vi "XML.ListElementTextValuesByCustomQuery.vi"(8 "error in":errorcluster, 10 "XPath expression":string, 11 "XML file path":path=path "C:/Projects/TM-OS/trunk/Design/XML_HW_config2.xml") -> (0 "error out":errorcluster, 2 "values":string[](array[string]))   [LabVIEW 2019, in "Tools.lvlib"]
uses:
  <vilib>/xml/Load XML File.vi
  <vilib>/xml/Close Reference(Node).vi
  Tools.lvlib
  <vilib>/xml/NI_XML.lvlib
  <resource>/objmgr/DOMUserDefRef.rc
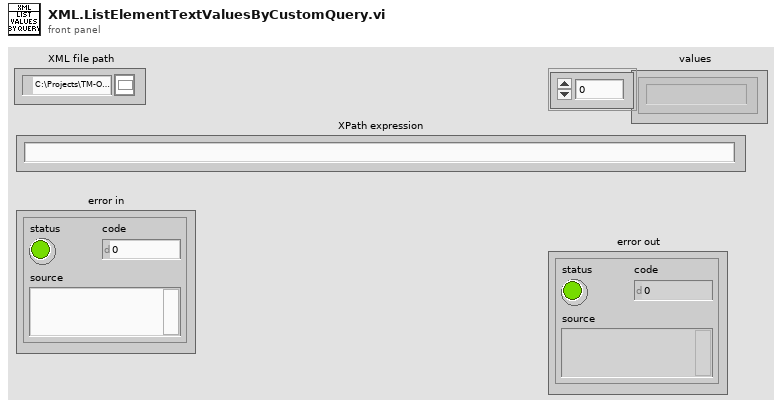
[diagram p1: front panel]
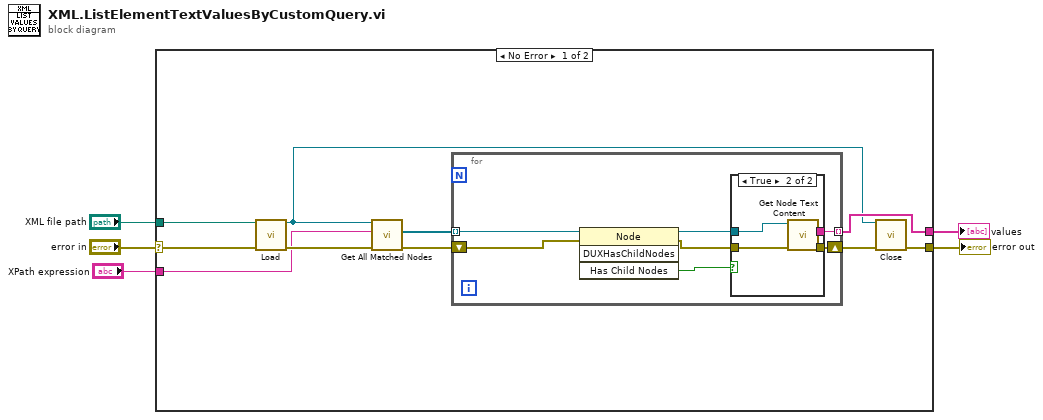
[diagram p0: block diagram]
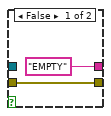
[diagram p2: hidden frame]
diagram:
  n1 = case shown="No Error" "error in" {
    selector: "error in" -> [w14 w29]
    tunnel: [w6 w29] -> w5
    tunnel: "XML file path" -> [w15 _]
    tunnel: [w11 _] -> w2
    tunnel: "XPath expression" -> [w9 _]
    frame No Error {
      n2 = call-poly <vilib>:"Load.vi"("path to XML document"=w15, "error in (no error)"=w14) -> ("DOM document out"=w8:refnum<k20>, "error out"=w10:errorcluster)  [unwired: 11 in, 1 out]
      n3 = call <vilib>:"Get All Matched Nodes.vi"("error in (no error)"=w10, "XPath expression"=w9, "node in"=w8) -> ("error out"=w12:errorcluster, "node result array"=w13:refnum<k20>[])  [unwired: 6 in, 1 out]
      n4 = for {
        tunnel: w13 -> [w17] mode=indexing
        tunnel: [w19] -> w11 mode=indexing
        shift-right: [w18] -> w7
        shift-left: w12 -> [w16]
        n5 = invoke class="Node" method="DUXHasChildNodes"(reference=w17, error in=w16) -> (reference out=w21:refnum<k20>, error out=w22:errorcluster, "Has Child Nodes"=w20:bool)  [unwired: 2 in, 1 out]
        n6 = case shown="True" w20 {
          tunnel: [w23 w28] -> w18
          tunnel: w22 -> [w23 w27]
          tunnel: w21 -> [_ w26]
          tunnel: ["EMPTY" w25] -> w19
          frame False {
          }
          frame True {
            n7 = call <vilib>:"Get Node Text Content.vi"("error in (no error)"=w27, "node in"=w26) -> ("error out"=w28:errorcluster, "node text"=w25:string)  [unwired: 7 in, 1 out]
          }
        }
      }
      n8 = call-poly <vilib>:"Close.vi"("error in (no error)"=w7, "node"=w8) -> ("error out"=w6:errorcluster)  [unwired: 7 in]
    }
    frame Error {
    }
  }
  "error out" <- w5
  "values" <- w2
